vi "headlights.vi"(7 "LabVIEW Web Service Request":refnum<class "Web Request.lvclass">, 11 "name":string) -> (3 "value":string)   [LabVIEW 2015]
uses:
  <vilib>/wsapi/Web Request.lvclass
  utilities/GlobalSender.vi
panel:
  # "Use the Web Service Request input terminal to call the VIs on the Web Services palette. Do not remove it from the connector pane unless you don't need access to the palette."
  # "Each additional control wired to the connector pane will be available as an input in the URL. To include an indicator in terminal-mode output (the default setting), it must also be wired to the connector pane."
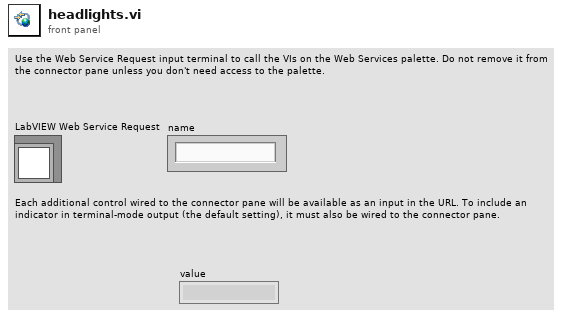
[diagram p1: front panel]
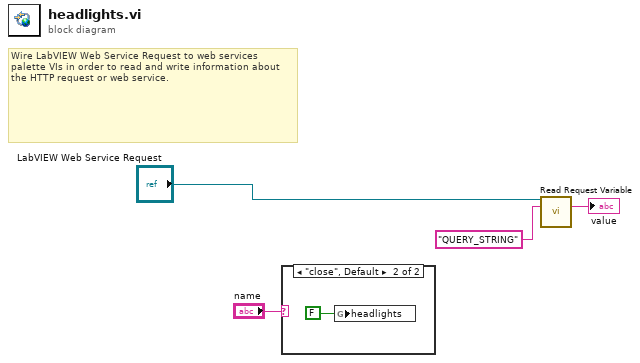
[diagram p0: block diagram]
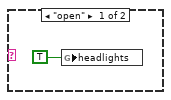
[diagram p2: hidden frame]
diagram:
  # "Wire LabVIEW Web Service Request to web services palette VIs in order to read and write information about the HTTP request or web service."
  n1 = case shown="\"close\", Default" "name" {
    frame "open" {
      n2 = global write "GlobalSender.vi" "headlights"(TRUE) -> ()
    }
    frame "close", Default {
      n3 = global write "GlobalSender.vi" "headlights"(FALSE) -> ()
    }
  }
  n4 = call <vilib>:"Read Request Variable.vi"("LabVIEW Web Service Request"="LabVIEW Web Service Request", "variable name"="QUERY_STRING") -> ("value"=→"value":string)  [unwired: 11 in, 2 out]
